vi "SendLogOutRequestEvent.vi"(8 "error in (no error)":errorcluster, 11 "TopLevel in":refnum<class "TopLevel.lvclass">) -> (0 "error out":errorcluster, 3 "TopLevel out":refnum<class "TopLevel.lvclass">)   [LabVIEW 2022 SP3, in "TopLevel.lvclass"]
uses:
  TopLevel.lvclass
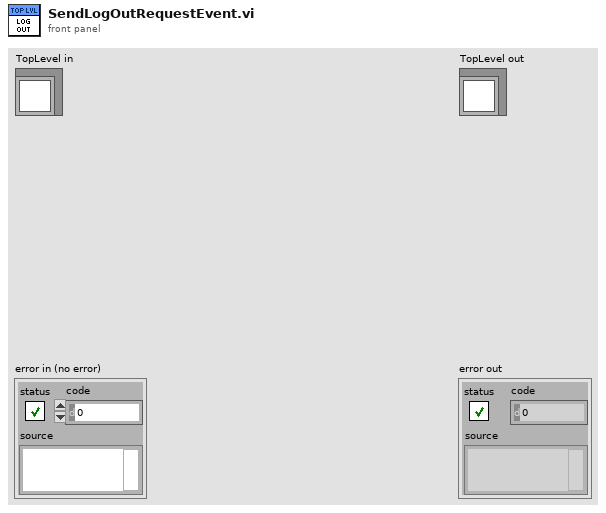
[diagram p1: front panel]
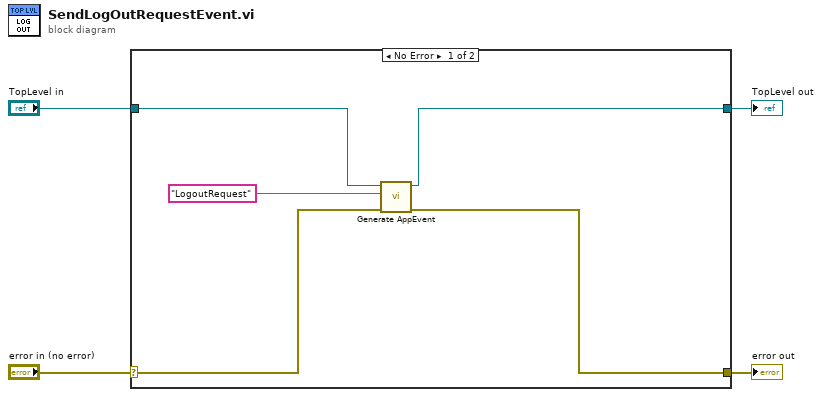
[diagram p0: block diagram]
diagram:
  n1 = case shown="No Error" "error in (no error)" {
    selector: "error in (no error)" -> [w7 w11]
    tunnel: [w6 w11] -> w3
    tunnel: [w9 w10] -> w1
    tunnel: "TopLevel in" -> [w8 w10]
    frame No Error {
      n2 = call-dynamic "Generate AppEvent.vi"("error in (no error)"=w7, "Command"="LogoutRequest", "TopLevel in"=w8) -> ("error out"=w6:errorcluster, "TopLevel out"=w9:refnum<class "TopLevel.lvclass">)  [unwired: 7 in]
    }
    frame Error {
    }
  }
  "error out" <- w3
  "TopLevel out" <- w1
